vi "20150719_Online_Program_emergency - 복사본.vi"() -> ()   [LabVIEW 2014]
uses:
  <vilib>/Utility/file.llb/Read From Spreadsheet File (DBL).vi
  <vilib>/Analysis/Matrix/Numeric/Conversions/Array To Matrix - RA2.vi
  <vilib>/Instr/_visa.llb/VISA Configure Serial Port (Instr).vi
  <vilib>/Analysis/Matrix/Numeric/Conversions/Array To Matrix - RA.vi
  <vilib>/Utility/file.llb/Write To Spreadsheet File (DBL).vi
  <vilib>/Utility/file.llb/Write To Spreadsheet File (I64).vi
  <vilib>/Analysis/Matrix/NI_Matrix.lvlib
  NeuroSky_Dll_Call/Debug/NeuroSky_Dll_Call.dll
  user32.dll
panel:
  out "에러 출력":errorcluster
  out "메시지 2":string
  out "큐사인":bool
  out "icon_온도":bool
  out "icon_용변":bool
  out "icon_자판":bool
  out "icon_응급":bool=TRUE
  out "icon_기계":bool
  out "icon_침대":bool
  out "메시지":string
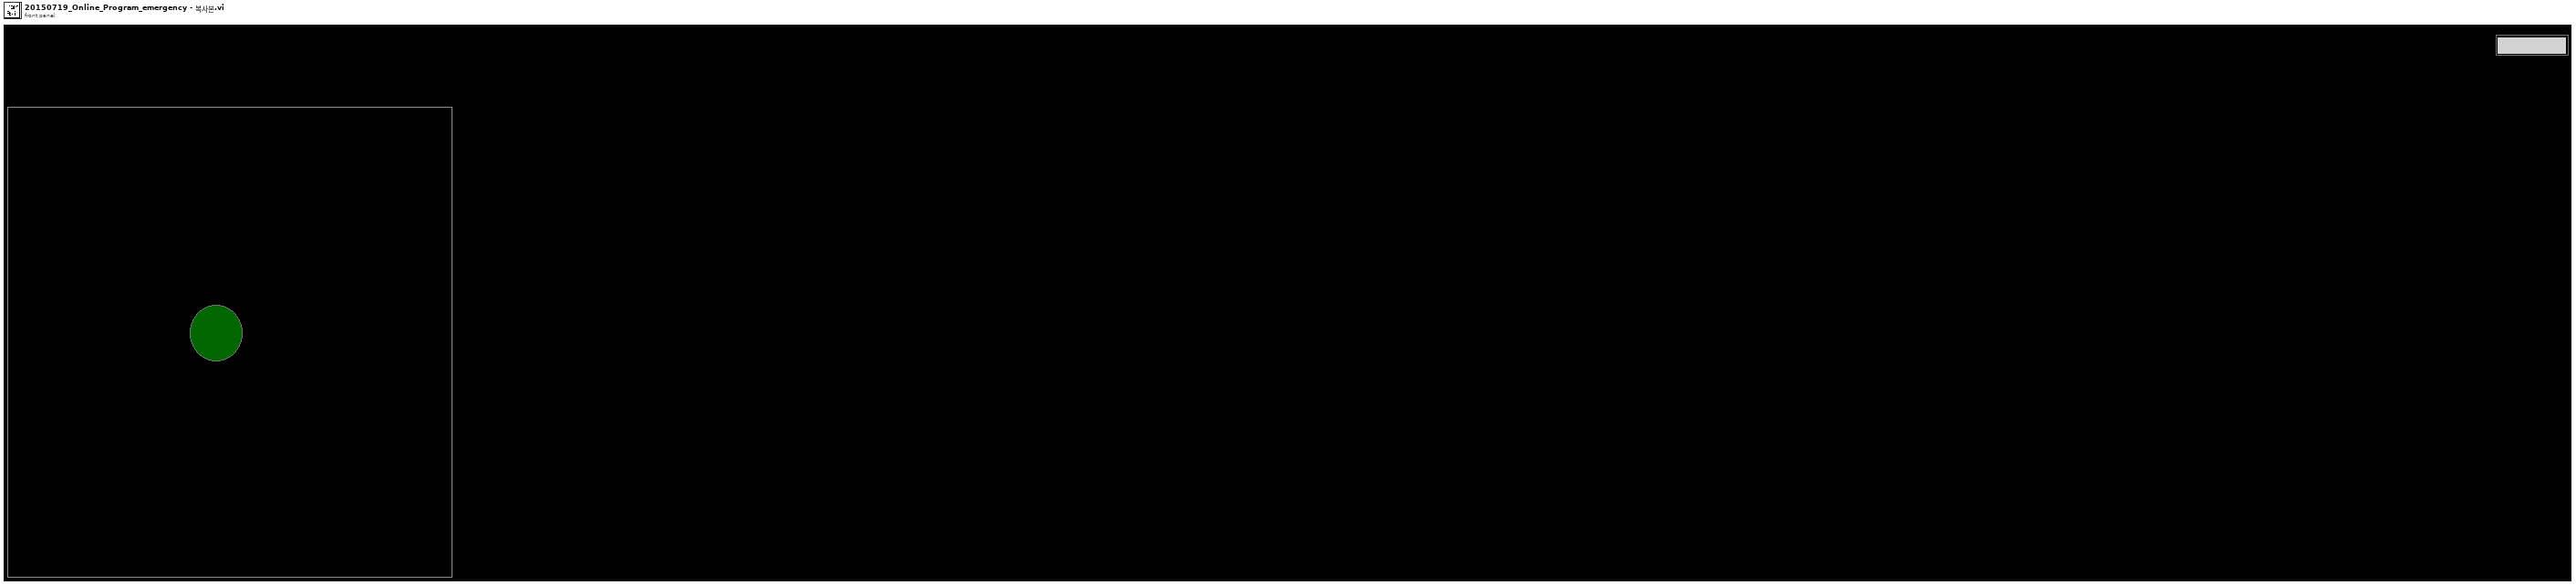
[diagram p1: front panel]
types:
  T1 = typedef "NI_Matrix.lvlib/RealMatrix.ctl" = dbl[][]
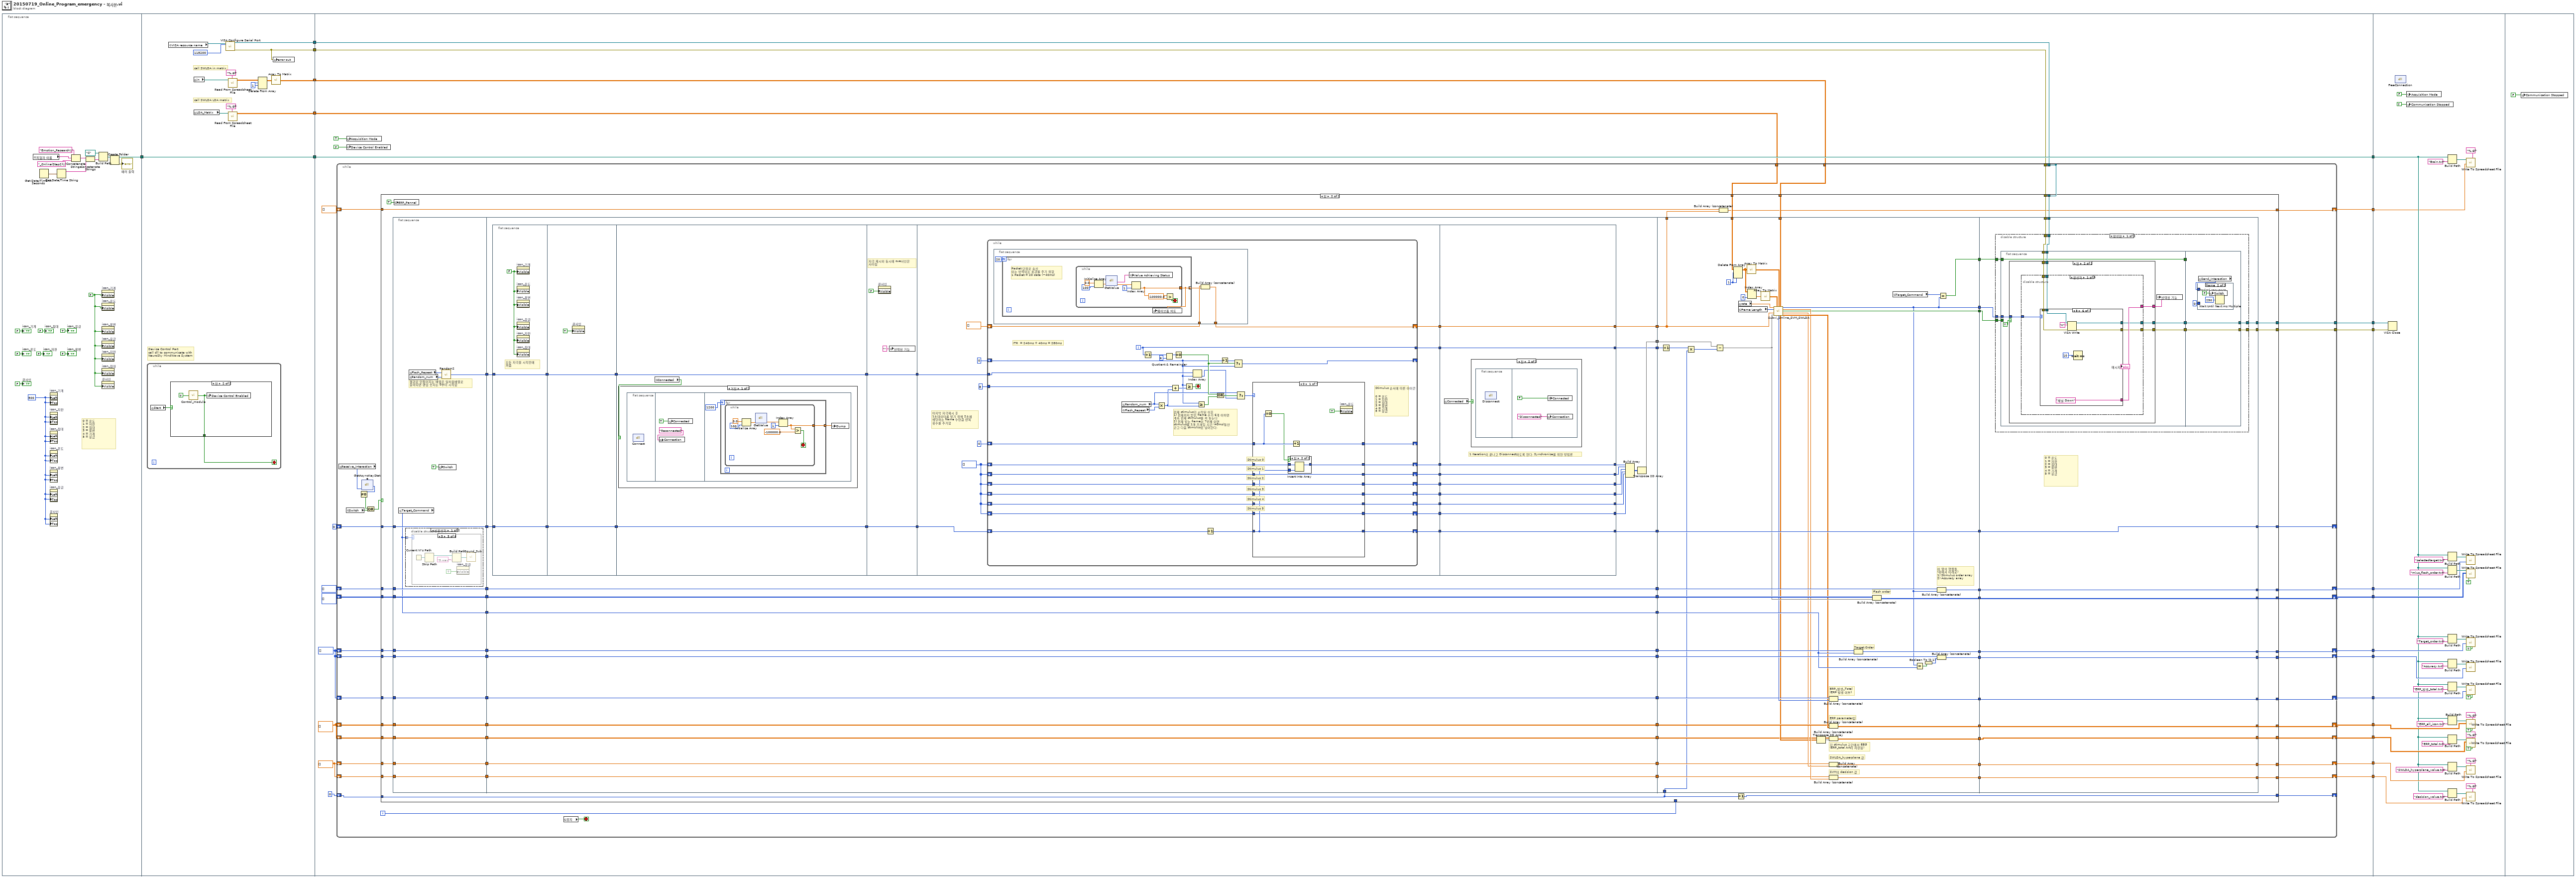
[diagram p0: block diagram]
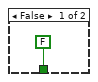
[diagram p2: hidden frame]
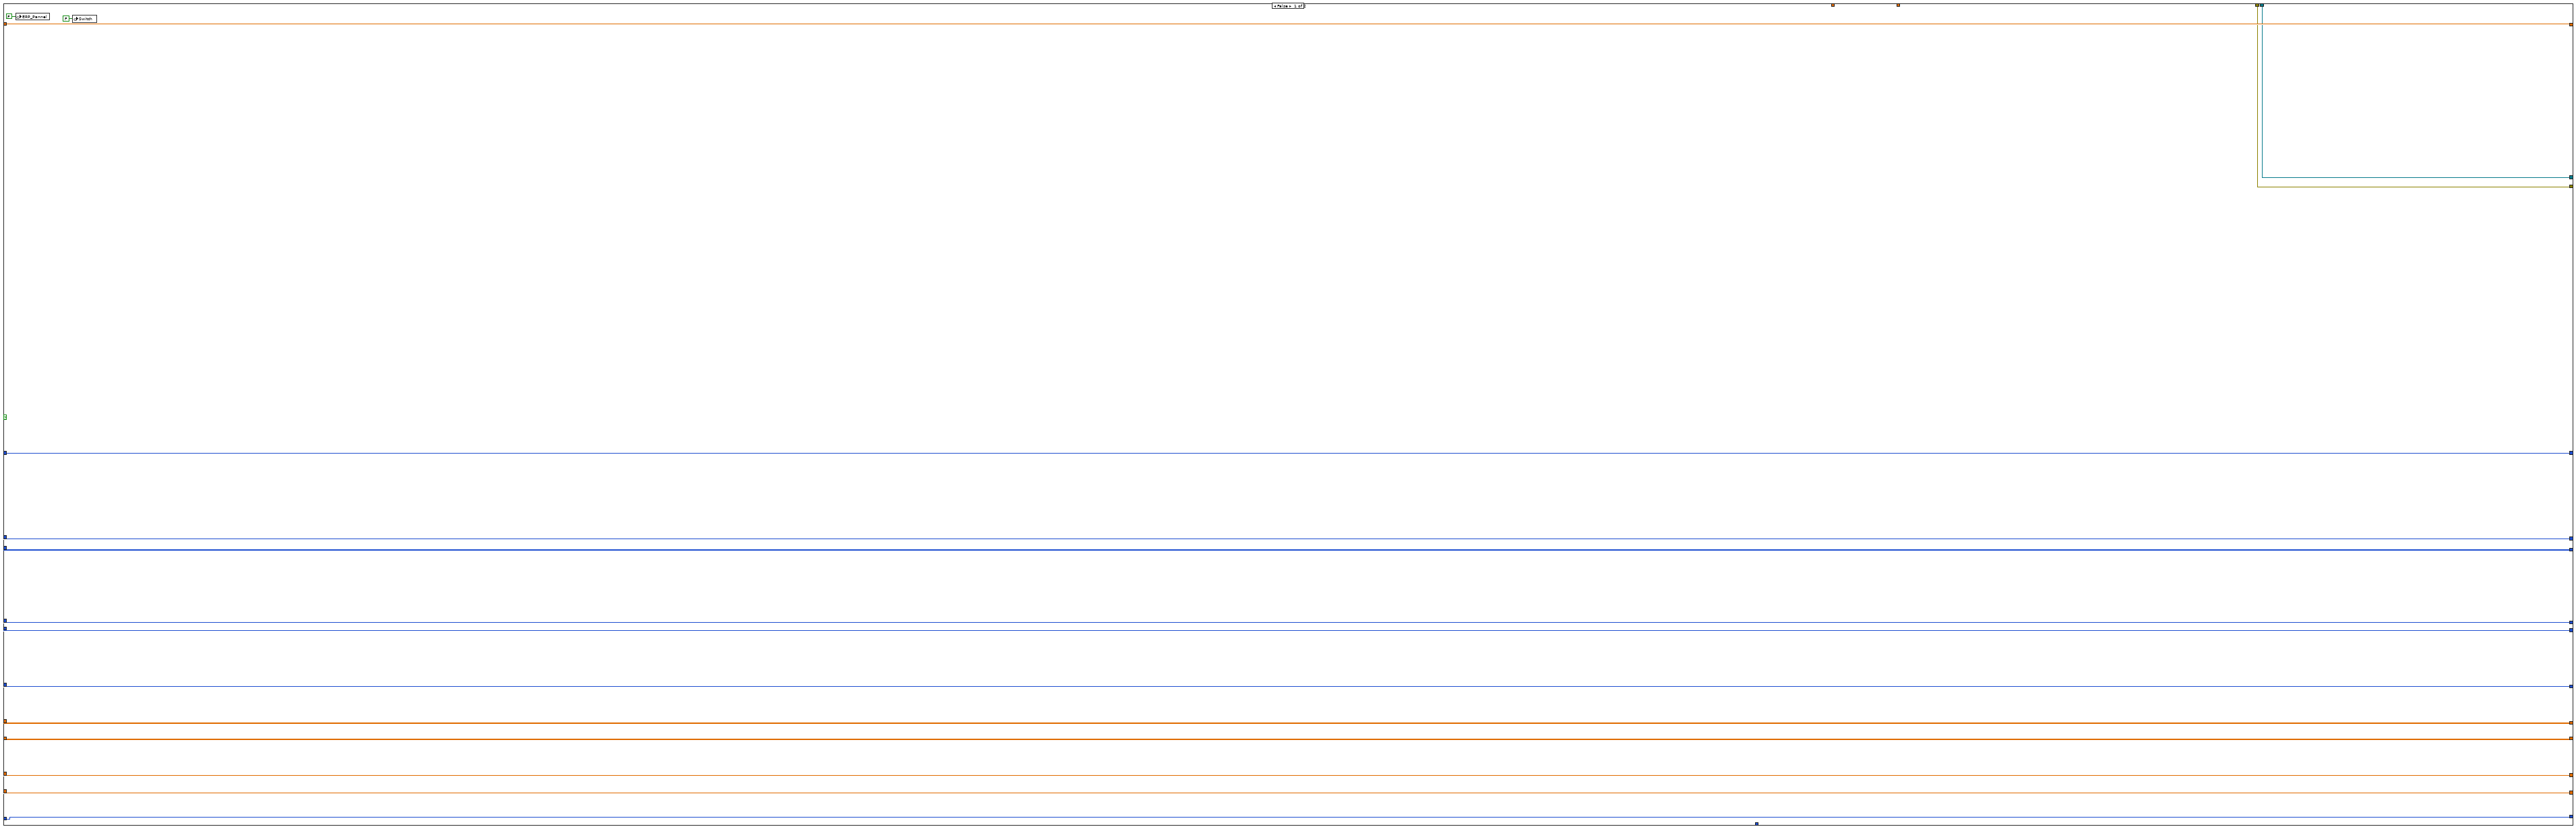
[diagram p3: hidden frame]
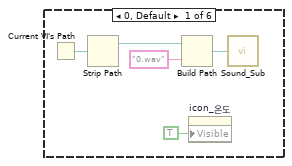
[diagram p4: hidden frame]
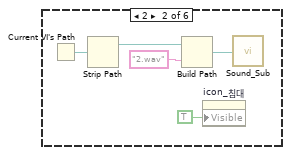
[diagram p5: hidden frame]
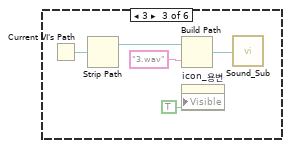
[diagram p6: hidden frame]
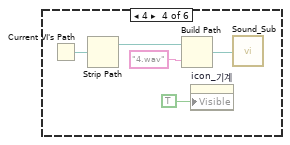
[diagram p7: hidden frame]
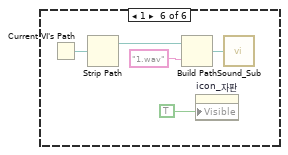
[diagram p8: hidden frame]
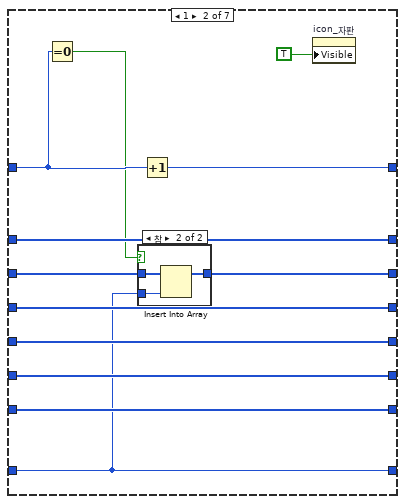
[diagram p12: hidden frame]
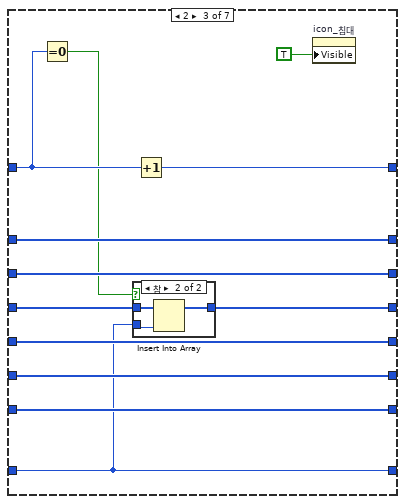
[diagram p14: hidden frame]
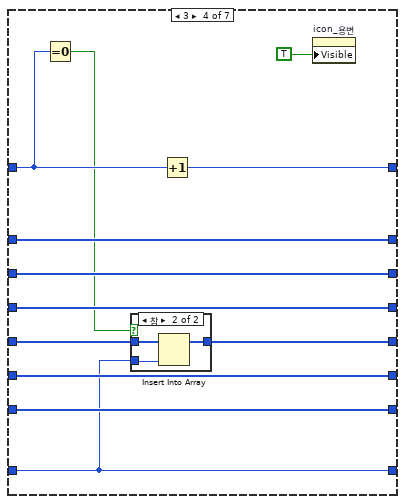
[diagram p16: hidden frame]
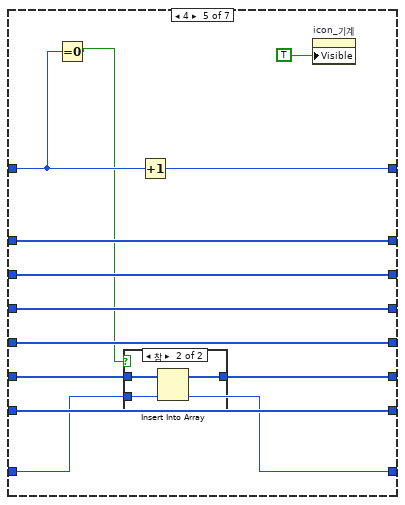
[diagram p18: hidden frame]
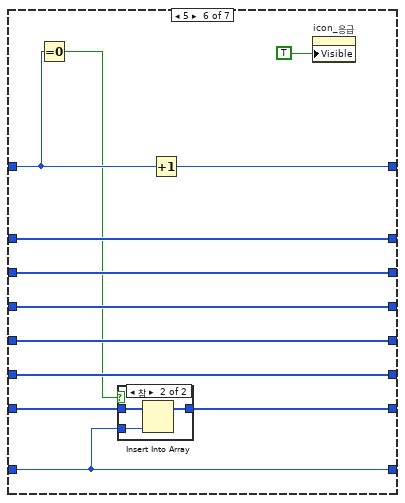
[diagram p20: hidden frame]
diagram:
  n1 = flat-sequence {
    tunnel: [w39] -> w19
    tunnel: w19 -> [w53]
    tunnel: [w53] -> w18
    tunnel: [w51] -> w17
    tunnel: [w44] -> w7
    tunnel: [w43] -> w4
    tunnel: [w42] -> w3
    tunnel: w18 -> [w76]
    tunnel: [w76] -> w16
    tunnel: [w85] -> w15
    tunnel: [w83] -> w14
    tunnel: [w81] -> w13
    tunnel: w17 -> [w66]
    tunnel: [w80] -> w12
    tunnel: [w77] -> w11
    tunnel: [w73] -> w10
    tunnel: [w72] -> w9
    tunnel: [w71] -> w8
    tunnel: w7 -> [w65]
    tunnel: [w69] -> w6
    tunnel: [w67] -> w5
    tunnel: w4 -> [w64]
    tunnel: w3 -> [w63]
    tunnel: [w62] -> w2
    tunnel: [w61] -> w1
    tunnel: w16 -> [w747]
    tunnel: w15 -> [w742]
    tunnel: w14 -> [w781]
    tunnel: w13 -> [w777]
    tunnel: w12 -> [w774]
    tunnel: w11 -> [w770]
    tunnel: w10 -> [w764]
    tunnel: w9 -> [w759]
    tunnel: w8 -> [w756]
    tunnel: w6 -> [w753]
    tunnel: w5 -> [w748]
    tunnel: w2 -> [w744]
    tunnel: w1 -> [w743]
    frame #0 {
      w20 = FALSE ("Visible")
      w22 = 500 ("Position:Left")
      # "0 = 온도\n1 = 자판\n2 = 침대\n3 = 용변 \n4 = 기계 \n5 = 응급"
      n2 = global read "Control_Panel_정리.vi" "피험자 이름"() -> (w30:string)
      n3 = Get Date/Time In Seconds() -> (seconds since 1Jan1904=w36:timestamp)
      n4 = property on="icon_기계" class="Bool (엄격한)"("Left"=w22, "Top"=w22) -> ()  [unwired: 2 in, 2 out]
      n5 = property on="icon_자판" class="Bool (엄격한)"("Left"=w22, "Top"=w22) -> ()  [unwired: 2 in, 2 out]
      n6 = property on="icon_침대" class="Bool (엄격한)"("Left"=w22, "Top"=w22) -> ()  [unwired: 2 in, 2 out]
      n7 = property on="icon_온도" class="Bool (엄격한)"("Left"=w22, "Top"=w22) -> ()  [unwired: 2 in, 2 out]
      n8 = property on="icon_용변" class="Bool (엄격한)"("Left"=w22, "Top"=w22) -> ()  [unwired: 2 in, 2 out]
      n9 = property on="icon_응급" class="Bool (엄격한)"("Left"=w22, "Top"=w22) -> ()  [unwired: 2 in, 2 out]
      n10 = property on="큐사인" class="Bool (엄격한)"("Left"=w22, "Top"=w22) -> ()  [unwired: 2 in, 2 out]
      n11 = Get Date/Time String(seconds (now)=w36) -> (date string=w37:string)  [unwired: 2 in, 1 out]
      n12 = Concatenate Strings("Emotion_Research\\" ("string"), w30, "_Online(Step2)\\" ("문자열")) -> (w32:string)
      n13 = Concatenate Strings(w32, w37) -> (w34:string)
      n14 = Build Path(base path=path "C:/" ("path"), name or relative path=w34) -> (appended path=w35:path)
      n15 = property on="icon_기계" class="Bool (엄격한)"("Visible"=w20) -> ()  [unwired: 2 in, 2 out]
      n16 = property on="icon_온도" class="Bool (엄격한)"("Visible"=w20) -> ()  [unwired: 2 in, 2 out]
      n17 = property on="icon_용변" class="Bool (엄격한)"("Visible"=w20) -> ()  [unwired: 2 in, 2 out]
      n18 = property on="icon_응급" class="Bool (엄격한)"("Visible"=w20) -> ()  [unwired: 2 in, 2 out]
      n19 = property on="icon_자판" class="Bool (엄격한)"("Visible"=w20) -> ()  [unwired: 2 in, 2 out]
      n20 = property on="icon_침대" class="Bool (엄격한)"("Visible"=w20) -> ()  [unwired: 2 in, 2 out]
      n21 = property on="큐사인" class="Bool (엄격한)"("Visible"=w20) -> ()  [unwired: 2 in, 2 out]
      n22 = Create Folder(path (use dialog)=w35) -> (created path=w39:path, error out=→"에러 출력":errorcluster)  [unwired: 2 in, 1 out]
      "icon_온도" <- FALSE ("icon_전원 6")
      "icon_용변" <- FALSE ("icon_전체종료")
      "icon_자판" <- FALSE ("icon_음량업 2")
      "icon_응급" <- TRUE ("icon_채널다운")
      "icon_기계" <- FALSE ("icon_음량다")
      "icon_침대" <- FALSE ("icon_채널업")
      "큐사인" <- FALSE ("icon_전원 7")
    }
    frame #1 {
      w47 = 1 ("인덱스 (행)")
      # "call SWLDA in matrix"
      # "call SWLDA LDA matrix"
      # "Device Control Part\ncall dll to communicate with\nNeuroSky MindWave System"
      n23 = while {
        stop <- w55 stop-if-true
        n24 = global read "Control_Panel_정리.vi" "Start"() -> (w54:bool)
        n25 = case shown="참" w54 {
          tunnel: [FALSE ("Connected") w57] -> w55
          frame False {
          }
          frame True {
            n26 = call "Control_module.vi"("Turn on"=TRUE ("Device Control Enabled")) -> ("Connected"=w57:bool)
            n27 = global write "Control_Panel_정리.vi" "Device Control Enabled"(w57) -> ()
          }
        }
      }
      n28 = global read "Control_Panel_정리.vi" "VISA resource name"() -> (w40:refnum<visa-resource-name>)
      n29 = global read "Control_Panel_정리.vi" "in"() -> (w45:path)
      n30 = global read "Control_Panel_정리.vi" "LDA_Matrix"() -> (w50:path)
      n31 = call-poly "VISA Configure Serial Port"("VISA resource name"=w40, "baud rate (9600)"=u32 115200) -> ("VISA resource name out"=w43:refnum<visa-resource-name>, "error out"=w42:errorcluster)  [unwired: 12 in]
      n32 = call-poly <vilib>:"Read From Spreadsheet File.vi"("format (%.3f)"="%.6f", "file path (dialog if empty)"=w45) -> ("all rows"=w46:dbl[][])  [unwired: 5 in, 4 out]
      n33 = call-poly <vilib>:"Read From Spreadsheet File.vi"("format (%.3f)"="%.6f", "file path (dialog if empty)"=w50) -> ("all rows"=w51:dbl[][])  [unwired: 5 in, 4 out]
      n34 = Delete From Array(array=w46, length=w47, index (row)=w47) -> (array with subset deleted=w48:dbl[][])  [unwired: 1 in, 1 out]
      n35 = call-poly <vilib>:"Array To Matrix.vi"("Real 2D Array"=w48) -> ("Real Matrix"=w44:T1)
      n36 = global write "Control_Panel_정리.vi" "error out"(w42) -> ()
    }
    frame #2 {
      w70 = dbl[] []
      w68 = dbl[][] []
      w60 = i16[] []
      n37 = while {
        shift-right: [w94] -> w85
        shift-left: dbl[] [] -> [w100]
        shift-right: [w121] -> _
        shift-left: 0 ("y") -> [w122]
        shift-right: [w115] -> w83
        shift-left: i32[][] [] -> [w116]
        shift-right: [w119] -> w81
        shift-left: i32[] [] -> [w120]
        shift-right: [w117] -> w80
        shift-left: w60 -> [w118]
        shift-right: [w112] -> w77
        shift-left: w60 -> [w113]
        shift-right: [w111] -> w73
        shift-left: w60 -> [w110]
        shift-right: [w109] -> w72
        shift-left: w68 -> [w108]
        shift-right: [w107] -> w71
        shift-left: w70 -> [w106]
        shift-right: [w105] -> w69
        shift-left: w70 -> [w104]
        shift-right: [w103] -> w67
        shift-left: w68 -> [w102]
        tunnel: w66 -> [w101]
        tunnel: w65 -> [w99]
        tunnel: [w97] -> _
        tunnel: w64 -> [w97]
        tunnel: w63 -> [w98]
        tunnel: [w96] -> w62
        tunnel: [w95] -> w61
        shift-right: [w88] -> _
        shift-left: 0 -> [w89]
        i -> [w114]
        stop <- w93 stop-if-true
        n38 = global read "Control_Panel_정리.vi" "Receive_Interaction"() -> (w91:u8)
        n39 = global read "Control_Panel_정리.vi" "Switch"() -> (w90:bool)
        n40 = dll-call lib="User32.dll" fn="GetAsyncKeyState"("vKey"=w91) -> ("return type"=w92:i64)  [unwired: 4 in, 2 out]
        n41 = Not Equal To 0?(x=w92) -> (x != 0?=w87:bool)
        n42 = Or(x=w87, y=w90) -> (x .or. y?=w86:bool)
        n43 = case shown="참" w86 {
          tunnel: w122 -> [w135 w172]
          tunnel: [w135 w171] -> w121
          tunnel: w120 -> [w134 w170]
          tunnel: [w134 w169] -> w119
          tunnel: w118 -> [w131 w168]
          tunnel: [w131 w167] -> w117
          tunnel: w116 -> [w133 w166]
          tunnel: [w133 w165] -> w115
          tunnel: w114 -> [_ _]
          tunnel: w113 -> [w132 w164]
          tunnel: [w132 w163] -> w112
          tunnel: [w130 w162] -> w111
          tunnel: w110 -> [w130 w161]
          tunnel: [w129 w160] -> w109
          tunnel: w108 -> [w129 w159]
          tunnel: [w127 w158] -> w107
          tunnel: w106 -> [w127 w157]
          tunnel: [w126 w156] -> w105
          tunnel: w104 -> [w126 w155]
          tunnel: [w128 w154] -> w103
          tunnel: w102 -> [w128 w153]
          tunnel: w101 -> [_ w152]
          tunnel: w100 -> [w138 w151]
          tunnel: w99 -> [_ w149]
          tunnel: w98 -> [w136 w148]
          tunnel: w97 -> [w137 w147]
          tunnel: [w137 w146] -> w96
          tunnel: [w136 w145] -> w95
          tunnel: [w138 w144] -> w94
          tunnel: w89 -> [w124 w140]
          tunnel: [w124 w139] -> w88
          frame False {
            n44 = global write "Control_Panel_정리.vi" "ERP_Pannel"(FALSE ("ERP_Pannel")) -> ()
            n45 = global write "Control_Panel_정리.vi" "Switch"(FALSE ("Switch")) -> ()
          }
          frame True {
            n46 = flat-sequence {
              tunnel: w172 -> [w224]
              tunnel: [w224] -> w209
              tunnel: [w214] -> w208
              tunnel: w170 -> [w223]
              tunnel: [w223] -> w207
              tunnel: w168 -> [w222]
              tunnel: [w222] -> w206
              tunnel: w166 -> [w221]
              tunnel: [w221] -> w205
              tunnel: [w220] -> w204
              tunnel: w164 -> [w220]
              tunnel: w161 -> [w219]
              tunnel: [w219] -> w203
              tunnel: w159 -> [w218]
              tunnel: [w218] -> w202
              tunnel: w157 -> [w217]
              tunnel: [w217] -> w201
              tunnel: w155 -> [w216]
              tunnel: [w216] -> w200
              tunnel: w153 -> [w215]
              tunnel: [w215] -> w199
              tunnel: [w210] -> w141
              tunnel: w209 -> [w293]
              tunnel: [w294] -> w198
              tunnel: [w283] -> w197
              tunnel: [w292] -> w196
              tunnel: [w291] -> w195
              tunnel: w208 -> [w290]
              tunnel: [w290] -> w194
              tunnel: w207 -> [w289]
              tunnel: [w289] -> w193
              tunnel: [w288] -> w192
              tunnel: w206 -> [w288]
              tunnel: [w287] -> w191
              tunnel: w205 -> [w287]
              tunnel: [w286] -> w190
              tunnel: w204 -> [w286]
              tunnel: [w285] -> w189
              tunnel: w203 -> [w285]
              tunnel: [w284] -> w188
              tunnel: w202 -> [w284]
              tunnel: [w282] -> w187
              tunnel: w201 -> [w282]
              tunnel: [w281] -> w186
              tunnel: w200 -> [w281]
              tunnel: w199 -> [w280]
              tunnel: [w280] -> w185
              tunnel: w141 -> [w259]
              tunnel: w198 -> [w539]
              tunnel: w197 -> [w513]
              tunnel: w196 -> [w551]
              tunnel: w195 -> [w552]
              tunnel: [w551] -> w174
              tunnel: [w511] -> w175
              tunnel: w194 -> [w538]
              tunnel: w193 -> [w547]
              tunnel: [w546] -> w176
              tunnel: w192 -> [w544]
              tunnel: [w543] -> w177
              tunnel: w191 -> [w542]
              tunnel: [w540] -> w178
              tunnel: w190 -> [w537]
              tunnel: [w536] -> w179
              tunnel: [w534] -> w180
              tunnel: w189 -> [w533]
              tunnel: [w531] -> w181
              tunnel: w188 -> [w530]
              tunnel: [w528] -> w182
              tunnel: w187 -> [w527]
              tunnel: [w525] -> w183
              tunnel: w186 -> [w524]
              tunnel: [w521] -> w184
              tunnel: w185 -> [w520]
              tunnel: w152 -> [w519]
              tunnel: [w513] -> w150
              tunnel: w149 -> [w515]
              tunnel: [w514] -> w173
              tunnel: [w510] -> w143
              tunnel: w140 -> [w509]
              tunnel: [w574] -> w171
              tunnel: [w573] -> w169
              tunnel: [w570] -> w167
              tunnel: [w572] -> w165
              tunnel: [w571] -> w163
              tunnel: [w569] -> w162
              tunnel: [w568] -> w160
              tunnel: [w567] -> w158
              tunnel: [w566] -> w156
              tunnel: [w565] -> w154
              tunnel: w184 -> [w565]
              tunnel: w183 -> [w566]
              tunnel: w182 -> [w567]
              tunnel: w181 -> [w568]
              tunnel: w180 -> [w569]
              tunnel: w179 -> [w571]
              tunnel: w178 -> [w572]
              tunnel: w177 -> [w570]
              tunnel: w176 -> [w573]
              tunnel: w175 -> [w564]
              tunnel: w174 -> [w574]
              tunnel: w173 -> [w563]
              tunnel: w148 -> [w562]
              tunnel: w147 -> [w561]
              tunnel: [w560] -> w146
              tunnel: [w559] -> w145
              tunnel: w143 -> [w558]
              frame #0 {
                # "결과로 만들어지는 배열은 일차원배열로\n출력되면 랜덤 숫자는 0부터 시작함"
                n47 = global read "Control_Panel_정리.vi" "Target_Command"() -> (w214:i32)
                n48 = disable-structure shown="비활성화" {
                  disable-tunnel: w214 -> [w225 _]
                  frame Disabled {
                    n49 = case shown="5" w225 {
                      frame 0, Default {
                        n50 = Current VI's Path() -> (path=w228:path)
                        n51 = Strip Path(path=w228) -> (stripped path=w229:path)  [unwired: 1 out]
                        n52 = Build Path(base path=w229, name or relative path="0.wav" ("이름 또는 상대 경로")) -> (appended path=w227:path)
                        n53 = property on="icon_온도" class="Bool (엄격한)"("Visible"=TRUE) -> ()  [unwired: 2 in, 2 out]
                        n54 = call "Sound_Sub.vi"("path"=w227) -> ()
                      }
                      frame 2 {
                        n55 = Current VI's Path() -> (path=w232:path)
                        n56 = Strip Path(path=w232) -> (stripped path=w233:path)  [unwired: 1 out]
                        n57 = Build Path(base path=w233, name or relative path="2.wav" ("이름 또는 상대 경로")) -> (appended path=w235:path)
                        n58 = property on="icon_침대" class="Bool (엄격한)"("Visible"=TRUE) -> ()  [unwired: 2 in, 2 out]
                        n59 = call "Sound_Sub.vi"("path"=w235) -> ()
                      }
                      frame 3 {
                        n60 = Current VI's Path() -> (path=w237:path)
                        n61 = Strip Path(path=w237) -> (stripped path=w238:path)  [unwired: 1 out]
                        n62 = Build Path(base path=w238, name or relative path="3.wav" ("이름 또는 상대 경로")) -> (appended path=w240:path)
                        n63 = property on="icon_용변" class="Bool (엄격한)"("Visible"=TRUE) -> ()  [unwired: 2 in, 2 out]
                        n64 = call "Sound_Sub.vi"("path"=w240) -> ()
                      }
                      frame 4 {
                        n65 = Current VI's Path() -> (path=w242:path)
                        n66 = Strip Path(path=w242) -> (stripped path=w243:path)  [unwired: 1 out]
                        n67 = Build Path(base path=w243, name or relative path="4.wav" ("이름 또는 상대 경로")) -> (appended path=w245:path)
                        n68 = property on="icon_기계" class="Bool (엄격한)"("Visible"=TRUE) -> ()  [unwired: 2 in, 2 out]
                        n69 = call "Sound_Sub.vi"("path"=w245) -> ()
                      }
                      frame 5 {
                        n70 = Current VI's Path() -> (path=w247:path)
                        n71 = Strip Path(path=w247) -> (stripped path=w248:path)  [unwired: 1 out]
                        n72 = Build Path(base path=w248, name or relative path="5.wav" ("이름 또는 상대 경로")) -> (appended path=w250:path)
                        n73 = property on="icon_응급" class="Bool (엄격한)"("Visible"=TRUE) -> ()  [unwired: 2 in, 2 out]
                        n74 = call "Sound_Sub.vi"("path"=w250) -> ()
                      }
                      frame 1 {
                        n75 = Current VI's Path() -> (path=w253:path)
                        n76 = Strip Path(path=w253) -> (stripped path=w254:path)  [unwired: 1 out]
                        n77 = Build Path(base path=w254, name or relative path="1.wav" ("이름 또는 상대 경로")) -> (appended path=w252:path)
                        n78 = property on="icon_자판" class="Bool (엄격한)"("Visible"=TRUE) -> ()  [unwired: 2 in, 2 out]
                        n79 = call "Sound_Sub.vi"("path"=w252) -> ()
                      }
                    }
                  }
                  frame Enabled {
                  }
                }
                n80 = global read "Control_Panel_정리.vi" "Flash_Repeat"() -> (w211:i32)
                n81 = global read "Control_Panel_정리.vi" "Random_num"() -> (w212:i32)
                n82 = global write "Control_Panel_정리.vi" "Switch"(TRUE ("Switch")) -> ()
                n83 = call "Random2.vi"("Random_num"=w212, "전체횟수"=w211) -> ("배열"=w210:i32[])
              }
              frame #1 {
                n84 = flat-sequence {
                  tunnel: w293 -> [w298]
                  tunnel: [w298] -> w279
                  tunnel: [w296] -> w260
                  tunnel: w259 -> [w296]
                  tunnel: [w301] -> w272
                  tunnel: w279 -> [w301]
                  tunnel: w260 -> [w299]
                  tunnel: [w299] -> w256
                  tunnel: w272 -> [w304]
                  tunnel: [w304] -> w262
                  tunnel: [w302] -> w257
                  tunnel: w256 -> [w302]
                  tunnel: w262 -> [w321]
                  tunnel: [w321] -> w261
                  tunnel: [w319] -> w258
                  tunnel: w257 -> [w319]
                  tunnel: w261 -> [w328]
                  tunnel: [w336] -> w271
                  tunnel: [w335] -> w270
                  tunnel: [w334] -> w269
                  tunnel: [w333] -> w268
                  tunnel: [w332] -> w267
                  tunnel: [w327] -> w266
                  tunnel: [w326] -> w265
                  tunnel: [w325] -> w264
                  tunnel: [w323] -> w263
                  tunnel: w258 -> [w322]
                  tunnel: [w498] -> w283
                  tunnel: [w499] -> w275
                  tunnel: [w500] -> w291
                  tunnel: [w501] -> w292
                  tunnel: [w502] -> w278
                  tunnel: [w503] -> w277
                  tunnel: [w504] -> w276
                  tunnel: [w505] -> w274
                  tunnel: [w506] -> w273
                  tunnel: w271 -> [w506]
                  tunnel: w270 -> [w505]
                  tunnel: w269 -> [w504]
                  tunnel: w268 -> [w503]
                  tunnel: w267 -> [w502]
                  tunnel: w266 -> [w501]
                  tunnel: w265 -> [w500]
                  tunnel: w264 -> [w499]
                  tunnel: w263 -> [w498]
                  frame #0 {
                    w297 = FALSE ("Visible")
                    # "모든 자극을 시작전에\n꺼줌"
                    n85 = property on="icon_기계" class="Bool (엄격한)"("Visible"=w297) -> ()  [unwired: 2 in, 2 out]
                    n86 = property on="icon_온도" class="Bool (엄격한)"("Visible"=w297) -> ()  [unwired: 2 in, 2 out]
                    n87 = property on="icon_용변" class="Bool (엄격한)"("Visible"=w297) -> ()  [unwired: 2 in, 2 out]
                    n88 = property on="icon_응급" class="Bool (엄격한)"("Visible"=w297) -> ()  [unwired: 2 in, 2 out]
                    n89 = property on="icon_자판" class="Bool (엄격한)"("Visible"=w297) -> ()  [unwired: 2 in, 2 out]
                    n90 = property on="icon_침대" class="Bool (엄격한)"("Visible"=w297) -> ()  [unwired: 2 in, 2 out]
                  }
                  frame #1 {
                    n91 = property on="큐사인" class="Bool (엄격한)"("Visible"=TRUE) -> ()  [unwired: 2 in, 2 out]
                  }
                  frame #2 {
                    n92 = global read "Control_Panel_정리.vi" "Connected"() -> (w303:bool)
                    n93 = case shown="거짓" w303 {
                      frame False {
                        n94 = flat-sequence {
                          frame #0 {
                            n95 = dll-call lib="C:/Users/Server/Desktop/NeuroSky/NeuroSky_Dll_Call/Debug/NeuroSky_Dll_Call.dll" fn="Connect"() -> ()  [unwired: 4 in, 2 out]
                          }
                          frame #1 {
                            n96 = global write "Control_Panel_정리.vi" "Connection"("Reconnected") -> ()
                            n97 = global write "Control_Panel_정리.vi" "Connected"(TRUE ("Connected")) -> ()
                          }
                          frame #2 {
                            n98 = for {
                              N: 1200 -> [_]
                              tunnel: [w309] -> w307 mode=indexing
                              n99 = while {
                                tunnel: [w311] -> w309
                                stop <- w310 stop-if-true
                                n100 = Initialize Array(0.0 ("element"), 100 ("dimension size")) -> (w316:dbl[])
                                n101 = dll-call lib="C:/Users/Server/Desktop/NeuroSky/NeuroSky_Dll_Call/Debug/NeuroSky_Dll_Call.dll" fn="GetValue"("result"=w316) -> ("result"=w317:dbl[])  [unwired: 4 in, 2 out]
                                n102 = Index Array(array=w317, index=1) -> (element=w311:dbl)
                                n103 = Greater?(x=w311, y=-100000.0) -> (0:w310:bool)
                              }
                            }
                            n104 = global write "Control_Panel_정리.vi" "Dump"(w307) -> ()
                          }
                        }
                      }
                      frame True {
                      }
                    }
                  }
                  frame #3 {
                    # "자극 제시와 동시에 cue사인은\n사라짐"
                    n105 = property on="큐사인" class="Bool (엄격한)"("Visible"=FALSE) -> ()  [unwired: 2 in, 2 out]
                    n106 = global write "Control_Panel_정리.vi" "선택된 기능"("" ("선택된 기능")) -> ()
                  }
                  frame #4 {
                    w330 = i32[] []
                    # "마지막 자극제시 후\n1초데이터를 받기 위해 2초에\n해당하는 frame 수만큼 반복\n횟수를 추가함"
                    n107 = while {
                      shift-right: [w344] -> w323
                      shift-left: dbl[] [] -> [w345]
                      tunnel: 8 -> [w341]
                      shift-right: [w371] -> w336
                      shift-left: w330 -> [w370]
                      shift-right: [w368] -> w335
                      shift-left: w330 -> [w369]
                      shift-right: [w366] -> w325
                      shift-left: w330 -> [w367]
                      shift-right: [w364] -> w334
                      shift-left: w330 -> [w365]
                      shift-right: [w362] -> w333
                      shift-left: w330 -> [w363]
                      shift-right: [w361] -> w332
                      shift-left: w330 -> [w349]
                      shift-right: [w359] -> w327
                      shift-left: w328 -> [w360]
                      shift-right: [w355] -> _
                      shift-left: 0 -> [w339]
                      shift-right: [w350] -> _
                      shift-left: 0 ("y") -> [w351]
                      tunnel: [w346] -> w326
                      tunnel: w322 -> [w340]
                      i -> [w346]
                      stop <- w374 stop-if-true
                      # "ITR  = 240ms + 40ms = 280ms"
                      # "현재 stimulus가 시작된 이후\n1) 현재까지 받은 frame 수가 6개 이하면\n계속 현재 stimulus를 켜 놓는다\n2) 현재 받는 frame이 7번째 이면\nstimulus를 1개 프레임 시간 (40ms)동안\n끈고 다음 stimulus로 넘어간다."
                      # "Stimulus 순서에 따른 아이콘\n\n\n0 = 온도\n1 = 자판\n2 = 침대\n3 = 용변 \n4 = 기계 \n5 = 응급"
                      # "Stimulus 5"
                      # "Stimulus 4"
                      # "Stimulus 3"
                      # "Stimulus 2"
                      # "Stimulus 1"
                      # "Stimulus 0"
                      n108 = flat-sequence {
                        tunnel: [w379] -> w344
                        tunnel: w345 -> [w378]
                        frame #0 {
                          n109 = for {
                            N: 20 -> [_]
                            tunnel: [w380] -> w377 mode=indexing
                            # "Packet 단위로 송신\n이는 반짝이는 효과를 주기 위함\n1 Packet = 20 data (~40ms)"
                            n110 = while {
                              tunnel: [w382] -> w380
                              stop <- w381 stop-if-true
                              n111 = Initialize Array(0.0 ("element"), 100 ("dimension size")) -> (w388:dbl[])
                              n112 = dll-call lib="C:/Users/Server/Desktop/NeuroSky/NeuroSky_Dll_Call/Debug/NeuroSky_Dll_Call.dll" fn="GetValue"("result"=w388) -> ("errCode"=w384:string, "result"=w389:dbl[])  [unwired: 3 in, 2 out]
                              n113 = global write "Control_Panel_정리.vi" "Value Achieving Status"(w384) -> ()
                              n114 = Index Array(array=w389, index=1) -> (element=w382:dbl)
                              n115 = Greater?(x=w382, y=-100000.0) -> (0:w381:bool)
                            }
                            n116 = global write "Control_Panel_정리.vi" "웨이브폼 차트"(w380) -> ()
                          }
                          n117 = Build Array (concatenate)(w378, w377) -> (w379:dbl[])
                        }
                      }
                      n118 = global read "Control_Panel_정리.vi" "Random_num"() -> (w343:i32)
                      n119 = global read "Control_Panel_정리.vi" "Flash_Repeat"() -> (w342:i32)
                      n120 = Increment(x=w346) -> (x+1=w348:i32)
                      n121 = Multiply(x=w343, y=w342) -> (x*y=w347:i32)
                      n122 = Quotient & Remainder(x=w348, y=6) -> (x-y*floor(x/y)=w357:i32)  [unwired: 1 out]
                      n123 = Add(x=w341, y=w347) -> (x+y=w375:i32)
                      n124 = Equal To 0?(x=w357) -> (x = 0?=w354:bool)
                      n125 = Greater Or Equal?(x=w339, y=w375) -> (x >= y?=w374:bool)
                      n126 = Index Array(array=w340, index=w339) -> (element=w338:i32)
                      n127 = Greater Or Equal?(x=w339, y=w347) -> (x >= y?=w353:bool)
                      n128 = Increment(x=w360) -> (x+1=w372:i32)
                      n129 = Or(x=w354, y=w353) -> (x .or. y?=w352:bool)
                      n130 = Increment(x=w339) -> (x+1=w356:i32)
                      n131 = Select(t=w356, s=w354, f=w339) -> (s? t:f=w355:i32)
                      n132 = Select(t=w343, s=w352, f=w338) -> (s? t:f=w373:i32)
                      n133 = case shown="0" w373 {
                        tunnel: w372 -> [w395 w411 w426 w442 w458 w475 w490]
                        tunnel: [w400 w408 w433 w449 w465 w481 w496] -> w371
                        tunnel: w370 -> [w401 w408 w433 w449 w465 w481 w496]
                        tunnel: w369 -> [w399 w417 w430 w446 w462 w479 w495]
                        tunnel: [w399 w416 w430 w446 w462 w479 w495] -> w368
                        tunnel: w367 -> [w398 w415 w432 w445 w461 w478 w494]
                        tunnel: [w398 w415 w431 w445 w461 w478 w494] -> w366
                        tunnel: w365 -> [w397 w414 w429 w448 w460 w477 w493]
                        tunnel: [w397 w414 w429 w447 w460 w477 w493] -> w364
                        tunnel: w363 -> [w396 w413 w428 w444 w464 w476 w492]
                        tunnel: [w396 w413 w428 w444 w463 w476 w492] -> w362
                        tunnel: w349 -> [w392 w412 w427 w443 w459 w480 w491]
                        tunnel: [w392 w412 w427 w443 w459 w472 w491] -> w361
                        tunnel: [w395 w411 w426 w442 w458 w475 w490] -> w359
                        tunnel: w351 -> [w394 w410 w425 w440 w457 w473 _]
                        tunnel: [w393 w409 w424 w441 w456 w474 0] -> w350
                        frame 0 {
                          n134 = Equal To 0?(x=w394) -> (x = 0?=w390:bool)
                          n135 = case shown="참" w390 {
                            tunnel: w401 -> [w402 w405]
                            tunnel: [w402 w404] -> w400
                            tunnel: w395 -> [_ w403]
                            frame False {
                            }
                            frame True {
                              n136 = Insert Into Array(array=w405, new element=w403) -> (w404:i32[])  [unwired: 1 in]
                            }
                          }
                          n137 = Increment(x=w394) -> (x+1=w393:i32)
                          n138 = property on="icon_온도" class="Bool (엄격한)"("Visible"=TRUE) -> ()  [unwired: 2 in, 2 out]
                        }
                        frame 1 {
                          n139 = Equal To 0?(x=w410) -> (x = 0?=w406:bool)
                          n140 = case shown="참" w406 {
                            tunnel: w417 -> [w418 w421]
                            tunnel: [w418 w420] -> w416
                            tunnel: w411 -> [_ w419]
                            frame False {
                            }
                            frame True {
                              n141 = Insert Into Array(array=w421, new element=w419) -> (w420:i32[])  [unwired: 1 in]
                            }
                          }
                          n142 = Increment(x=w410) -> (x+1=w409:i32)
                          n143 = property on="icon_자판" class="Bool (엄격한)"("Visible"=TRUE) -> ()  [unwired: 2 in, 2 out]
                        }
                        frame 2 {
                          n144 = Equal To 0?(x=w425) -> (x = 0?=w422:bool)
                          n145 = case shown="참" w422 {
                            tunnel: w432 -> [w434 w437]
                            tunnel: [w434 w436] -> w431
                            tunnel: w426 -> [_ w435]
                            frame False {
                            }
                            frame True {
                              n146 = Insert Into Array(array=w437, new element=w435) -> (w436:i32[])  [unwired: 1 in]
                            }
                          }
                          n147 = Increment(x=w425) -> (x+1=w424:i32)
                          n148 = property on="icon_침대" class="Bool (엄격한)"("Visible"=TRUE) -> ()  [unwired: 2 in, 2 out]
                        }
                        frame 3 {
                          n149 = Equal To 0?(x=w440) -> (x = 0?=w438:bool)
                          n150 = case shown="참" w438 {
                            tunnel: w448 -> [w450 w453]
                            tunnel: [w450 w452] -> w447
                            tunnel: w442 -> [_ w451]
                            frame False {
                            }
                            frame True {
                              n151 = Insert Into Array(array=w453, new element=w451) -> (w452:i32[])  [unwired: 1 in]
                            }
                          }
                          n152 = Increment(x=w440) -> (x+1=w441:i32)
                          n153 = property on="icon_용변" class="Bool (엄격한)"("Visible"=TRUE) -> ()  [unwired: 2 in, 2 out]
                        }
                        frame 4 {
                          n154 = Equal To 0?(x=w457) -> (x = 0?=w454:bool)
                          n155 = case shown="참" w454 {
                            tunnel: w464 -> [w466 w469]
                            tunnel: [w466 w468] -> w463
                            tunnel: w458 -> [_ w467]
                            frame False {
                            }
                            frame True {
                              n156 = Insert Into Array(array=w469, new element=w467) -> (w468:i32[])  [unwired: 1 in]
                            }
                          }
                          n157 = Increment(x=w457) -> (x+1=w456:i32)
                          n158 = property on="icon_기계" class="Bool (엄격한)"("Visible"=TRUE) -> ()  [unwired: 2 in, 2 out]
                        }
                        frame 5 {
                          n159 = Equal To 0?(x=w473) -> (x = 0?=w470:bool)
                          n160 = case shown="참" w470 {
                            tunnel: w480 -> [w482 w485]
                            tunnel: [w482 w484] -> w472
                            tunnel: w475 -> [_ w483]
                            frame False {
                            }
                            frame True {
                              n161 = Insert Into Array(array=w485, new element=w483) -> (w484:i32[])  [unwired: 1 in]
                            }
                          }
                          n162 = Increment(x=w473) -> (x+1=w474:i32)
                          n163 = property on="icon_응급" class="Bool (엄격한)"("Visible"=TRUE) -> ()  [unwired: 2 in, 2 out]
                        }
                        frame 6, Default {
                          w487 = FALSE ("Visible")
                          w488 = FALSE ("Visible")
                          w486 = FALSE ("Visible")
                          n164 = property on="icon_기계" class="Bool (엄격한)"("Visible"=w486) -> ()  [unwired: 2 in, 2 out]
                          n165 = property on="icon_온도" class="Bool (엄격한)"("Visible"=w486) -> ()  [unwired: 2 in, 2 out]
                          n166 = property on="icon_응급" class="Bool (엄격한)"("Visible"=w488) -> ()  [unwired: 2 in, 2 out]
                          n167 = property on="icon_용변" class="Bool (엄격한)"("Visible"=w488) -> ()  [unwired: 2 in, 2 out]
                          n168 = property on="icon_자판" class="Bool (엄격한)"("Visible"=w487) -> ()  [unwired: 2 in, 2 out]
                          n169 = property on="icon_침대" class="Bool (엄격한)"("Visible"=w487) -> ()  [unwired: 2 in, 2 out]
                        }
                      }
                    }
                  }
                  frame #5 {
                    # "1 Iteration이 끝나고 Disconnect하도록 한다. Synchronize를 위한 방법론"
                    n170 = global read "Control_Panel_정리.vi" "Connected"() -> (w497:bool)
                    n171 = case shown="참" w497 {
                      frame False {
                      }
                      frame True {
                        n172 = flat-sequence {
                          frame #0 {
                            n173 = dll-call lib="C:/Users/Server/Desktop/NeuroSky/NeuroSky_Dll_Call/Debug/NeuroSky_Dll_Call.dll" fn="Disconnect"() -> ()  [unwired: 4 in, 2 out]
                          }
                          frame #1 {
                            n174 = global write "Control_Panel_정리.vi" "Connection"("Disconnected") -> ()
                            n175 = global write "Control_Panel_정리.vi" "Connected"(FALSE ("Connected")) -> ()
                          }
                        }
                      }
                    }
                  }
                }
                n176 = Build Array(w273, w274, w275, w276, w277, w278) -> (w295:i32[][])
                n177 = Transpose 2D Array(2D array=w295) -> (transposed array=w294:i32[][])
              }
              frame #2 {
                w555 = 1 ("인덱스 (행)")
                # "각 stimulus 구간에서 EEG\n(ERP_total.txt라 저장됨)"
                # "ERP parameter값"
                # "SVM의 decision 값"
                # "SWLDA_hyperplane 값"
                # "ERP_발생_Total\n(ERP 발생 여부)"
                # "Target Order"
                # "Flash order"
                # "이 열의 행렬들 \n(위에서 아래로)\n1) Stimulus order array\n2) Accuracy array"
                n178 = Increment(x=w552) -> (x+1=w556:i32)
                n179 = Multiply(x=w556, y=w509) -> (x*y=w557:i32)
                n180 = Subtract(x=w539, y=w557) -> (x-y=w541:i32[][])
                n181 = Delete From Array(array=w519, length=w555, index (row)=w555) -> (array with subset deleted=w517:dbl[][])  [unwired: 1 in, 1 out]
                n182 = global read "Control_Panel_정리.vi" "rate"() -> (w549:dbl)
                n183 = global read "Control_Panel_정리.vi" "Frame Length"() -> (w550:i32)
                n184 = call-poly <vilib>:"Array To Matrix.vi"("Real 2D Array"=w517) -> ("Real Matrix"=w516:T1)
                n185 = Index Array(array=w517, index (col)=0 ("인덱스")) -> (element=w518:dbl[])  [unwired: 1 in]
                n186 = call-poly <vilib>:"Array To Matrix.vi"("Real 1D Array"=w518) -> ("Real Matrix (Column Vector)"=w553:T1)
                n187 = call "Subvi_Online_SVM_SWLDA.vi"("rate"=w549, "Value"=w553, "Matrix"=w516, "in"=w515, "samples per channel"=w550, "Brain_data_source"=w513, "Target_Flash_Order"=w541) -> ("output-0~8"=w511:i32, "decision"=w526:dbl[], "ERP_발생여부"=w514:bool, "SWLDA"=w529:dbl[], "EPR_발생_total"=w535:i16[], "ERP_all"=w523:dbl[][], "ERP_Parameters"=w532:dbl[][])  [unwired: 2 in]
                n188 = Transpose 2D Array(2D array=w523) -> (transposed array=w522:dbl[][])
                n189 = Build Array (concatenate)(w533, w535) -> (w534:i16[])
                n190 = Build Array (concatenate)(w530, w532) -> (w531:dbl[][])
                n191 = Build Array (concatenate)(w520, w522) -> (w521:dbl[][])
                n192 = Build Array (concatenate)(w527, w529) -> (w528:dbl[])
                n193 = Build Array (concatenate)(w524, w526) -> (w525:dbl[])
                n194 = Build Array (concatenate)(w537, w538) -> (w536:i32[])
                n195 = Build Array (concatenate)(w542, w541) -> (w540:i32[][])
                n196 = global read "Control_Panel_정리.vi" "Target_Command"() -> (w512:i32)
                n197 = Equal?(x=w511, y=w538) -> (x = y?=w548:bool)
                n198 = Boolean To (0,1)(Boolean=w548) -> (0, 1=w545:i16)
                n199 = Build Array (concatenate)(w547, w511) -> (w546:i32[])
                n200 = Build Array (concatenate)(w544, w545) -> (w543:i16[])
                n201 = Equal?(x=w512, y=w511) -> (x = y?=w510:bool)
              }
              frame #3 {
                # "0 = 온도\n1 = 자판\n2 = 침대\n3 = 용변 \n4 = 기계 \n5 = 응급"
                n202 = disable-structure shown="활성화" {
                  disable-tunnel: w564 -> [w584 w689]
                  disable-tunnel: w563 -> [w583 w688]
                  disable-tunnel: w562 -> [w582 _]
                  disable-tunnel: w561 -> [w581 _]
                  disable-tunnel: [w580 _] -> w560
                  disable-tunnel: [w579 _] -> w559
                  disable-tunnel: w558 -> [w576 w686]
                  frame Enabled {
                    n203 = flat-sequence {
                      tunnel: w584 -> [w592]
                      tunnel: w583 -> [_]
                      tunnel: w582 -> [w591]
                      tunnel: w581 -> [w590]
                      tunnel: [w589] -> w578
                      tunnel: [w588] -> w577
                      tunnel: w576 -> [w586]
                      tunnel: [w586] -> w575
                      tunnel: [w677] -> w579
                      tunnel: [w678] -> w580
                      tunnel: w578 -> [w678]
                      tunnel: w577 -> [w677]
                      tunnel: w575 -> [_]
                      frame #0 {
                        n204 = case shown="참" TRUE {
                          tunnel: w592 -> [_ w601]
                          tunnel: ["No Decesion" ("메시지") w600] -> w587
                          tunnel: w591 -> [w593 w599]
                          tunnel: w590 -> [w594 w598]
                          tunnel: [w594 w597] -> w589
                          tunnel: [w593 w596] -> w588
                          frame False {
                          }
                          frame True {
                            n205 = disable-structure shown="활성화" {
                              disable-tunnel: [w607 _ "" ("메시지")] -> w600
                              disable-tunnel: w601 -> [w602 w649 _]
                              disable-tunnel: w599 -> [w606 _ _]
                              disable-tunnel: w598 -> [w605 _ _]
                              disable-tunnel: [w604 _ _] -> w597
                              disable-tunnel: [w603 _ _] -> w596
                              frame Enabled {
                                n206 = case shown="5" w602 {
                                tunnel: ["전원" ("메시지") "음향 UP" ("메시지") "채널 UP" ("메시지") "전체종료" ("메시지") "음향 Down" ("메시지") "채널 Down" ("메시지") "No Decesion" ("메시지")] -> w607
                                tunnel: w606 -> [w611 w618 w624 w629 w635 w642 w646]
                                tunnel: w605 -> [w610 w617 w625 w630 w634 w641 w647]
                                tunnel: [w609 w616 w623 w630 w633 w640 w647] -> w604
                                tunnel: [w608 w615 w622 w629 w632 w639 w646] -> w603
                                frame 0 {
                                n207 = VISA Write(VISA resource name=w610, write buffer="0", error in (no error)=w611) -> (VISA resource name out=w609:refnum<visa-resource-name>, error out=w608:errorcluster)  [unwired: 1 out]
                                n208 = Wait (ms)(milliseconds to wait=u32 10) -> ()  [unwired: 1 out]
                                }
                                frame 1 {
                                n209 = VISA Write(VISA resource name=w617, write buffer="L", error in (no error)=w618) -> (VISA resource name out=w616:refnum<visa-resource-name>, error out=w615:errorcluster)  [unwired: 1 out]
                                n210 = Wait (ms)(milliseconds to wait=u32 10) -> ()  [unwired: 1 out]
                                }
                                frame 2 {
                                n211 = VISA Write(VISA resource name=w625, write buffer="J", error in (no error)=w624) -> (VISA resource name out=w623:refnum<visa-resource-name>, error out=w622:errorcluster)  [unwired: 1 out]
                                n212 = Wait (ms)(milliseconds to wait=u32 10) -> ()  [unwired: 1 out]
                                }
                                frame 3 {
                                }
                                frame 4 {
                                n213 = VISA Write(VISA resource name=w634, write buffer="M", error in (no error)=w635) -> (VISA resource name out=w633:refnum<visa-resource-name>, error out=w632:errorcluster)  [unwired: 1 out]
                                n214 = Wait (ms)(milliseconds to wait=u32 10) -> ()  [unwired: 1 out]
                                }
                                frame 5 {
                                n215 = VISA Write(VISA resource name=w641, write buffer="K", error in (no error)=w642) -> (VISA resource name out=w640:refnum<visa-resource-name>, error out=w639:errorcluster)  [unwired: 1 out]
                                n216 = Wait (ms)(milliseconds to wait=u32 10) -> ()  [unwired: 1 out]
                                }
                                frame 9, Default {
                                }
                                }
                              }
                              frame Disabled {
                                n217 = case shown="0, 기본" w649 {
                                frame 0, Default {
                                n218 = Current VI's Path() -> (path=w651:path)
                                n219 = Strip Path(path=w651) -> (stripped path=w652:path)  [unwired: 1 out]
                                n220 = Build Path(base path=w652, name or relative path="0.wav" ("이름 또는 상대 경로")) -> (appended path=w650:path)
                                n221 = call "Sound_Sub.vi"("path"=w650) -> ()
                                }
                                frame 2 {
                                n222 = Current VI's Path() -> (path=w654:path)
                                n223 = Strip Path(path=w654) -> (stripped path=w655:path)  [unwired: 1 out]
                                n224 = Build Path(base path=w655, name or relative path="2.wav" ("이름 또는 상대 경로")) -> (appended path=w657:path)
                                n225 = call "Sound_Sub.vi"("path"=w657) -> ()
                                }
                                frame 3 {
                                n226 = Current VI's Path() -> (path=w658:path)
                                n227 = Strip Path(path=w658) -> (stripped path=w659:path)  [unwired: 1 out]
                                n228 = Build Path(base path=w659, name or relative path="3.wav" ("이름 또는 상대 경로")) -> (appended path=w661:path)
                                n229 = call "Sound_Sub.vi"("path"=w661) -> ()
                                }
                                frame 4 {
                                n230 = Current VI's Path() -> (path=w662:path)
                                n231 = Strip Path(path=w662) -> (stripped path=w663:path)  [unwired: 1 out]
                                n232 = Build Path(base path=w663, name or relative path="4.wav" ("이름 또는 상대 경로")) -> (appended path=w665:path)
                                n233 = call "Sound_Sub.vi"("path"=w665) -> ()
                                }
                                frame 5 {
                                n234 = Current VI's Path() -> (path=w666:path)
                                n235 = Strip Path(path=w666) -> (stripped path=w667:path)  [unwired: 1 out]
                                n236 = Build Path(base path=w667, name or relative path="5.wav" ("이름 또는 상대 경로")) -> (appended path=w669:path)
                                n237 = call "Sound_Sub.vi"("path"=w669) -> ()
                                }
                                frame 1 {
                                n238 = Current VI's Path() -> (path=w671:path)
                                n239 = Strip Path(path=w671) -> (stripped path=w672:path)  [unwired: 1 out]
                                n240 = Build Path(base path=w672, name or relative path="1.wav" ("이름 또는 상대 경로")) -> (appended path=w670:path)
                                n241 = call "Sound_Sub.vi"("path"=w670) -> ()
                                }
                                }
                              }
                              frame Disabled {
                              }
                            }
                          }
                        }
                        n242 = global write "Control_Panel_정리.vi" "선택된 기능"(w587) -> ()
                      }
                      frame #1 {
                        n243 = global read "Control_Panel_정리.vi" "Send_Interaction"() -> (w676:u8)
                        n244 = stacked-sequence {
                          tunnel: w676 -> [w680 _ w685]
                          tunnel: u32 0 ("dwFlags") -> [w679 _ w684]
                          frame #0 {
                            n245 = dll-call lib="User32.dll" fn="keybd_event"("bVk"=w680, "bScan"=w679, "dwFlags"=w679, "dwExtraInfo"=w679) -> ()  [unwired: 8 in, 2 out]
                          }
                          frame #1 {
                            n246 = global write "Control_Panel_정리.vi" "Switch"(FALSE ("Switch")) -> ()
                            n247 = Wait Until Next ms Multiple(millisecond multiple=u32 250) -> ()  [unwired: 1 out]
                          }
                          frame #2 {
                            n248 = dll-call lib="User32.dll" fn="keybd_event"("bVk"=w685, "bScan"=w684, "dwFlags"=u32 2, "dwExtraInfo"=w684) -> ()  [unwired: 8 in, 2 out]
                          }
                        }
                      }
                    }
                  }
                  frame Disabled {
                    n249 = flat-sequence {
                      tunnel: w689 -> [w693]
                      tunnel: w688 -> [w692]
                      tunnel: [w690] -> w687
                      tunnel: w686 -> [w690]
                      tunnel: w687 -> [w732]
                      frame #0 {
                        n250 = case shown="참" w692 {
                          tunnel: w693 -> [_ w696]
                          tunnel: ["No Decesion" ("메시지") w695] -> w691
                          frame False {
                          }
                          frame True {
                            n251 = disable-structure shown="활성화" {
                              disable-tunnel: [w698 _ "" ("메시지")] -> w695
                              disable-tunnel: w696 -> [w697 w706 _]
                              frame Enabled {
                                n252 = case shown="4" w697 {
                                tunnel: ["온도" ("메시지") "자판" ("메시지") "침대" ("메시지") "용변" ("메시지") "기계" ("메시지") "응급" ("메시지") "No Decesion" ("메시지")] -> w698
                                frame 0 {
                                }
                                frame 1 {
                                }
                                frame 2 {
                                }
                                frame 3 {
                                }
                                frame 4 {
                                }
                                frame 5 {
                                }
                                frame 9, Default {
                                }
                                }
                              }
                              frame Disabled {
                                n253 = case shown="4" w706 {
                                frame 0, Default {
                                n254 = Current VI's Path() -> (path=w708:path)
                                n255 = Strip Path(path=w708) -> (stripped path=w709:path)  [unwired: 1 out]
                                n256 = Build Path(base path=w709, name or relative path="0.wav" ("이름 또는 상대 경로")) -> (appended path=w707:path)
                                n257 = call "Sound_Sub.vi"("path"=w707) -> ()
                                }
                                frame 2 {
                                n258 = Current VI's Path() -> (path=w711:path)
                                n259 = Strip Path(path=w711) -> (stripped path=w712:path)  [unwired: 1 out]
                                n260 = Build Path(base path=w712, name or relative path="2.wav" ("이름 또는 상대 경로")) -> (appended path=w714:path)
                                n261 = call "Sound_Sub.vi"("path"=w714) -> ()
                                }
                                frame 3 {
                                n262 = Current VI's Path() -> (path=w715:path)
                                n263 = Strip Path(path=w715) -> (stripped path=w716:path)  [unwired: 1 out]
                                n264 = Build Path(base path=w716, name or relative path="3.wav" ("이름 또는 상대 경로")) -> (appended path=w718:path)
                                n265 = call "Sound_Sub.vi"("path"=w718) -> ()
                                }
                                frame 4 {
                                n266 = Current VI's Path() -> (path=w719:path)
                                n267 = Strip Path(path=w719) -> (stripped path=w720:path)  [unwired: 1 out]
                                n268 = Build Path(base path=w720, name or relative path="4.wav" ("이름 또는 상대 경로")) -> (appended path=w722:path)
                                n269 = call "Sound_Sub.vi"("path"=w722) -> ()
                                }
                                frame 5 {
                                n270 = Current VI's Path() -> (path=w723:path)
                                n271 = Strip Path(path=w723) -> (stripped path=w724:path)  [unwired: 1 out]
                                n272 = Build Path(base path=w724, name or relative path="5.wav" ("이름 또는 상대 경로")) -> (appended path=w726:path)
                                n273 = call "Sound_Sub.vi"("path"=w726) -> ()
                                }
                                frame 1 {
                                n274 = Current VI's Path() -> (path=w728:path)
                                n275 = Strip Path(path=w728) -> (stripped path=w729:path)  [unwired: 1 out]
                                n276 = Build Path(base path=w729, name or relative path="1.wav" ("이름 또는 상대 경로")) -> (appended path=w727:path)
                                n277 = call "Sound_Sub.vi"("path"=w727) -> ()
                                }
                                }
                              }
                              frame Disabled {
                              }
                            }
                          }
                        }
                        n278 = global write "Control_Panel_정리.vi" "선택된 기능"(w691) -> ()
                      }
                      frame #1 {
                        n279 = case shown="참" w732 {
                          frame False {
                          }
                          frame True {
                            n280 = global read "Control_Panel_정리.vi" "Send_Interaction"() -> (w735:u8)
                            n281 = stacked-sequence {
                              tunnel: w735 -> [w737 _ w741]
                              tunnel: u32 0 ("dwFlags") -> [w736 _ w740]
                              frame #0 {
                                n282 = dll-call lib="User32.dll" fn="keybd_event"("bVk"=w737, "bScan"=w736, "dwFlags"=w736, "dwExtraInfo"=w736) -> ()  [unwired: 8 in, 2 out]
                              }
                              frame #1 {
                                n283 = Wait Until Next ms Multiple(millisecond multiple=u32 250) -> ()  [unwired: 1 out]
                              }
                              frame #2 {
                                n284 = dll-call lib="User32.dll" fn="keybd_event"("bVk"=w741, "bScan"=w740, "dwFlags"=u32 2, "dwExtraInfo"=w740) -> ()  [unwired: 8 in, 2 out]
                              }
                            }
                            n285 = global write "Control_Panel_정리.vi" "Switch"(FALSE ("Switch")) -> ()
                          }
                        }
                      }
                    }
                  }
                }
              }
            }
            n286 = global write "Control_Panel_정리.vi" "ERP_Pannel"(TRUE ("ERP_Pannel")) -> ()
            n287 = Build Array (concatenate)(w151, w150) -> (w144:dbl[])
            n288 = Increment(x=w140) -> (x+1=w139:i32)
          }
        }
        n289 = global read "Control_Panel_정리.vi" "정지"() -> (w93:bool)
      }
      n290 = global write "Control_Panel_정리.vi" "Acquisition Mode"(TRUE ("Device Control Enabled")) -> ()
      n291 = global write "Control_Panel_정리.vi" "Device Control Enabled"(FALSE ("Device Control Enabled")) -> ()
    }
    frame #3 {
      n292 = VISA Close(VISA resource name=w744, error in (no error)=w743) -> ()  [unwired: 1 out]
      n293 = dll-call lib="C:/Users/Server/Desktop/NeuroSky/NeuroSky_Dll_Call/Debug/NeuroSky_Dll_Call.dll" fn="FreeConnection"() -> ()  [unwired: 4 in, 2 out]
      n294 = global write "Control_Panel_정리.vi" "Acquisition Mode"(FALSE ("Device Control Enabled")) -> ()
      n295 = global write "Control_Panel_정리.vi" "Communication Stopped"(TRUE ("Device Control Enabled")) -> ()
      n296 = Build Path(base path=w747, name or relative path="Brain.txt") -> (appended path=w786:path)
      n297 = Build Path(base path=w747, name or relative path="selectedtarget.txt") -> (appended path=w778:path)
      n298 = Build Path(base path=w747, name or relative path="mius_flash_order.txt") -> (appended path=w783:path)
      n299 = Build Path(base path=w747, name or relative path="Target_order.txt") -> (appended path=w773:path)
      n300 = Build Path(base path=w747, name or relative path="Accuracy.txt") -> (appended path=w776:path)
      n301 = Build Path(base path=w747, name or relative path="ERP_발생_total.txt") -> (appended path=w766:path)
      n302 = Build Path(base path=w747, name or relative path="ERP_all_icon.txt") -> (appended path=w762:path)
      n303 = Build Path(base path=w747, name or relative path="ERP_total.txt") -> (appended path=w750:path)
      n304 = Build Path(base path=w747, name or relative path="SWLDA_hyperplane_value.txt") -> (appended path=w758:path)
      n305 = Build Path(base path=w747, name or relative path="decision_value.txt") -> (appended path=w755:path)
      n306 = call-poly <vilib>:"Write To Spreadsheet File.vi"("format (%.3f)"="%.6f", "1D data"=w742, "file path (dialog if empty)"=w786) -> ()  [unwired: 5 in, 1 out]
      n307 = call-poly <vilib>:"Write To Spreadsheet File.vi"("1D data"=w777, "file path (dialog if empty)"=w778) -> ()  [unwired: 6 in, 1 out]
      n308 = call-poly <vilib>:"Write To Spreadsheet File.vi"("transpose? (no:F)"=TRUE, "2D data"=w781, "file path (dialog if empty)"=w783) -> ()  [unwired: 5 in, 1 out]
      n309 = call-poly <vilib>:"Write To Spreadsheet File.vi"("transpose? (no:F)"=TRUE, "1D data"=w770, "file path (dialog if empty)"=w773) -> ()  [unwired: 5 in, 1 out]
      n310 = call-poly <vilib>:"Write To Spreadsheet File.vi"("1D data"=w774, "file path (dialog if empty)"=w776) -> ()  [unwired: 6 in, 1 out]
      n311 = call-poly <vilib>:"Write To Spreadsheet File.vi"("transpose? (no:F)"=TRUE, "1D data"=w764, "file path (dialog if empty)"=w766) -> ()  [unwired: 5 in, 1 out]
      n312 = call-poly <vilib>:"Write To Spreadsheet File.vi"("transpose? (no:F)"=TRUE, "format (%.3f)"="%.6f", "2D data"=w759, "file path (dialog if empty)"=w762) -> ()  [unwired: 4 in, 1 out]
      n313 = call-poly <vilib>:"Write To Spreadsheet File.vi"("transpose? (no:F)"=TRUE, "format (%.3f)"="%.6f", "2D data"=w748, "file path (dialog if empty)"=w750) -> ()  [unwired: 4 in, 1 out]
      n314 = call-poly <vilib>:"Write To Spreadsheet File.vi"("format (%.3f)"="%.6f", "1D data"=w756, "file path (dialog if empty)"=w758) -> ()  [unwired: 5 in, 1 out]
      n315 = call-poly <vilib>:"Write To Spreadsheet File.vi"("format (%.3f)"="%.6f", "1D data"=w753, "file path (dialog if empty)"=w755) -> ()  [unwired: 5 in, 1 out]
    }
    frame #4 {
      n316 = global write "Control_Panel_정리.vi" "Communication Stopped"(FALSE ("Device Control Enabled")) -> ()
    }
  }
